vi "importSessionFluorophore.vi"(8 "error in (no error)":errorcluster, 10 "Clust Refnum":refnum<vi>, 11 "Database in":refnum<class "Database.lvclass">) -> (0 "error out":errorcluster, 2 "Clust Refnum 2":refnum<vi>, 3 "Database out":refnum<class "Database.lvclass">)   [LabVIEW 2014, in "Database.lvclass"]
uses:
  Database.lvclass
  Database.lvclass/Database.ctl
  <vilib>/addons/database/NI_Database_API.lvlib
panel:
  in  "session__fluorophore":T1
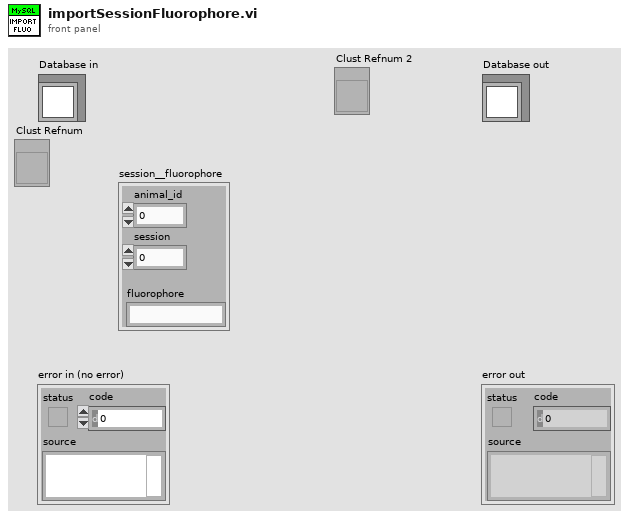
[diagram p1: front panel]
types:
  T1 = cluster{"animal_id":dbl, "session":dbl, "fluorophore":string}
  T2 = typedef "NI_Database_API.lvlib/Conn ObjectReference.ctl" = refnum<k1>
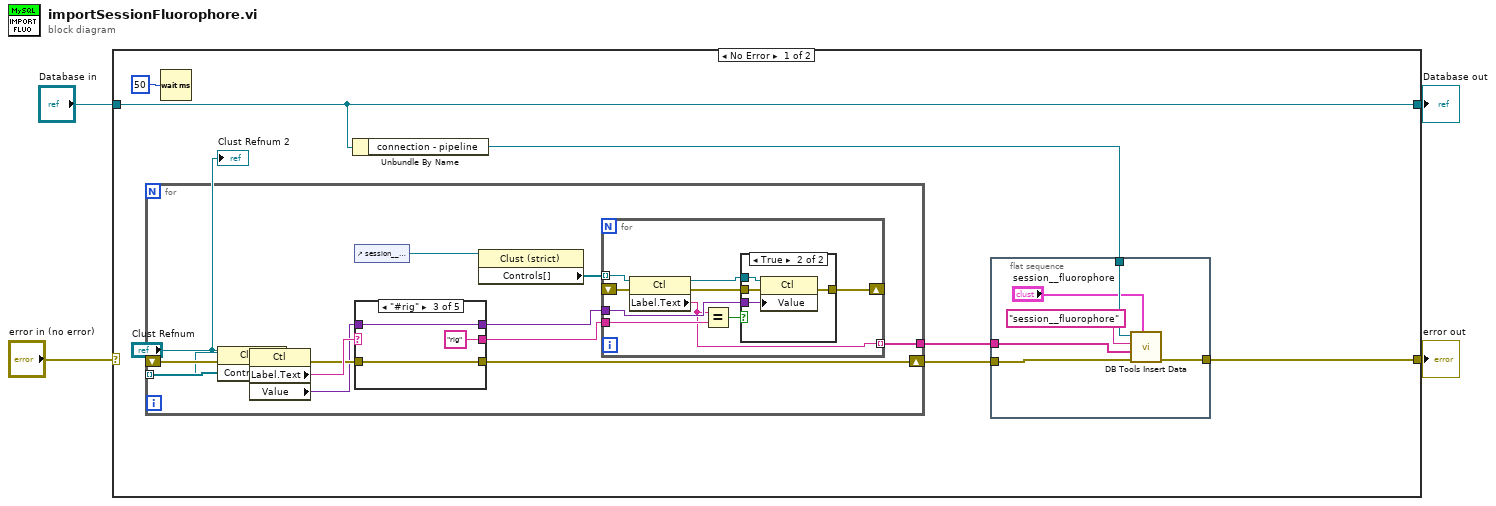
[diagram p0: block diagram]
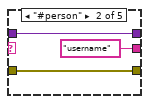
[diagram p4: hidden frame]
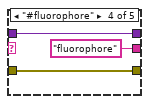
[diagram p5: hidden frame]
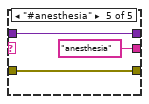
[diagram p6: hidden frame]
diagram:
  n1 = case shown="No Error" "error in (no error)" {
    selector: "error in (no error)" -> [_ w61]
    tunnel: [w7 w61] -> w3
    tunnel: [w9 w60] -> w1
    tunnel: "Database in" -> [w9 w60]
    frame No Error {
      n2 = Wait (ms)(milliseconds to wait=u32 50) -> ()  [unwired: 1 out]
      n3 = property class="Clust"(reference="Clust Refnum") -> (error out=w12:errorcluster, "Controls[]"=w13:refnum<vi>[])  [unwired: 1 in, 1 out]
      n4 = for {
        tunnel: w13 -> [w30] mode=indexing
        shift-right: [w20] -> w8
        shift-left: w12 -> [w29]
        tunnel: [w22] -> w11
        n5 = property class="Ctl"(reference=w30, error in=w29) -> (error out=w27:errorcluster, "Label.Text"=w28:string, "Value"=w26:variant)  [unwired: 1 out]
        n6 = control-ref of="session__fluorophore"() -> (w21:refnum<vi>)
        n7 = case shown="\"#rig\"" w28 {
          selector: w28 -> [w47 _ _ _ _]
          tunnel: [w47 "username" ("session") "rig" ("session") "fluorophore" ("session") "anesthesia"] -> w23
          tunnel: w27 -> [w46 w48 w51 w55 w58]
          tunnel: [w46 w48 w51 w55 w58] -> w20
          tunnel: w26 -> [w45 w49 w52 w54 w57]
          tunnel: [w45 w49 w52 w54 w57] -> w24
          frame "False", Default {
          }
          frame "#person" {
          }
          frame "#rig" {
          }
          frame "#fluorophore" {
          }
          frame "#anesthesia" {
          }
        }
        n8 = property class="Clust (strict)"(reference=w21) -> ("Controls[]"=w25:refnum<vi>[])  [unwired: 1 in, 2 out]
        n9 = for {
          tunnel: w23 -> [w39]
          tunnel: w24 -> [w36]
          tunnel: w25 -> [w38] mode=indexing
          tunnel: [w34] -> w22 mode=indexing
          shift-right: [w31] -> _
          shift-left: _ -> [w33]
          n10 = property class="Ctl"(reference=w38, error in=w33) -> (reference out=w37:refnum<vi>, error out=w32:errorcluster, "Label.Text"=w34:string)
          n11 = Equal?(x=w34, y=w39) -> (x = y?=w35:bool)
          n12 = case shown="True" w35 {
            tunnel: w37 -> [_ w44]
            tunnel: w36 -> [_ w43]
            tunnel: w32 -> [w40 w42]
            tunnel: [w40 w41] -> w31
            frame False {
            }
            frame True {
              n13 = property class="Ctl"(reference=w44, error in=w42, "Value"=w43) -> (error out=w41:errorcluster)  [unwired: 1 out]
            }
          }
        }
      }
      n14 = Unbundle By Name(w9) -> ("connection - pipeline"=w6:T2)
      n15 = flat-sequence {
        tunnel: w11 -> [w19]
        tunnel: w8 -> [w17]
        tunnel: [w16] -> w7
        tunnel: w6 -> [w15]
        frame #0 {
          n16 = call <vilib>:"DB Tools Insert Data.vi"("data"="session__fluorophore", "error in (no error)"=w17, "columns"=w19, "table"="session__fluorophore" ("session"), "connection reference"=w15) -> ("error out"=w16:errorcluster)  [unwired: 5 in, 1 out]
        }
      }
      "Clust Refnum 2" <- "Clust Refnum"
    }
    frame Error {
    }
  }
  "error out" <- w3
  "Database out" <- w1
